vi "Coral Teleop Handler.vi"() -> ()   [LabVIEW 2023]
uses:
  Teleop Util/Coral States.ctl
  Teleop Util/Scoring Setpoint.ctl
  Teleop Util/Scoring Levels.ctl
  <vilib>/Rock Robotics/WPI/Joystick/XBox Axes Indexer.ctl
  <vilib>/Rock Robotics/WPI/Joystick/XBox Buttons Indexer.ctl
  Coral/Implementation/Coral Operations.ctl
  02b96f5f-4aa0-4050-af39-5bf6ce57af74.vi
  ac154037-dd92-4d3b-9487-38ca34f15abd.vi
  41f243a3-b476-470d-886f-9ab9dadf628b.vi
  d73daf83-586d-4580-b12c-c6ead0d00ab0.vi
  <vilib>/Rock Robotics/WPI/Utilities/WPI_GetSetVariantRefNum.vi
  Framework/Robot Global Data.vi
panel:
  in  "Left Rumble":sgl
  out "Final Setpoint":T1=enum."L2"
  in  "Scoring Setpoint":T2=[enum."Trough", enum."L2", enum."L3", enum."L4"]
  out "testing states bz":T3
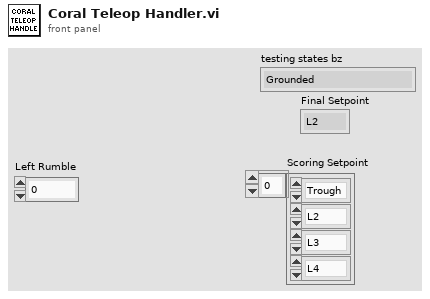
[diagram p1: front panel]
types:
  T1 = typedef "Scoring Levels.ctl" = enum16{"Trough", "L2", "L3", "L4", "Default"}
  T2 = typedef "Scoring Setpoint.ctl" = enum16{"Trough", "L2", "L3", "L4"}[]
  T3 = typedef "Coral States.ctl" = enum16{"Grounded", "Coral Intake", "Scoring Sequence", "Hold Position", "Score", "Manual Override", "Climb Safety Mode"}
  T4 = typedef "XBox Buttons Indexer.ctl" = enum16{"A", "B", "X", "Y", "Left Bumper", "Right Bumper", "Back", "Start", "Left Joystick", "Right Joystick"}
  T5 = typedef "XBox Axes Indexer.ctl" = enum16{"Left X", "Left Y", "Left Trigger", "Right Trigger", "Right X", "Right Y"}
  T6 = typedef "WPI_JoystickDevRef.ctl" = cluster{"Device":T7}
  T7 = typedef "WPI_JoystickDeviceEnum.ctl" = enum16{"USB 0", "USB 1", "USB 2", "USB 3", "USB 4", "USB 5"}
  T8 = typedef "Coral Operations.ctl" = enum16{"Reserve", "Read Current", "Immediate", "Calibrate"}
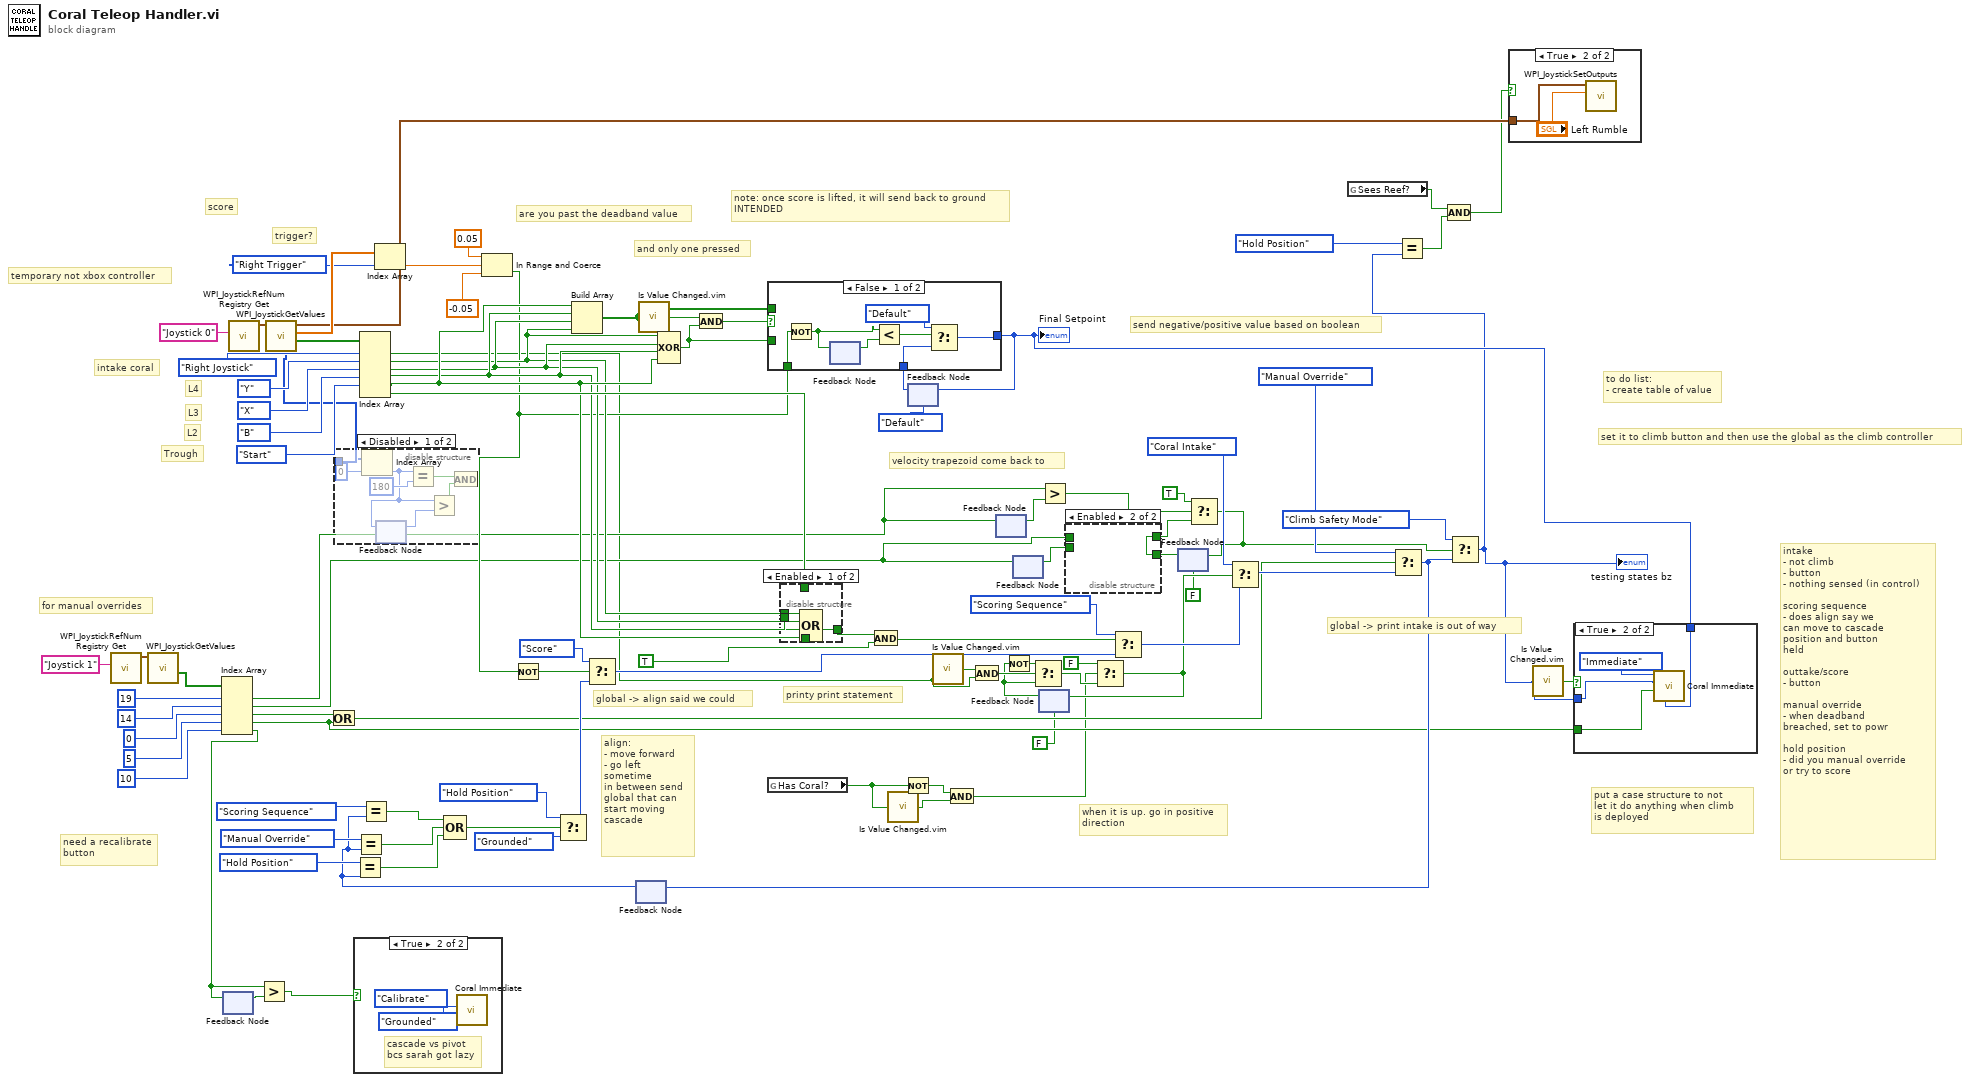
[diagram p0: block diagram]
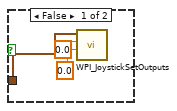
[diagram p2: hidden frame]
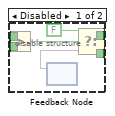
[diagram p4: hidden frame]
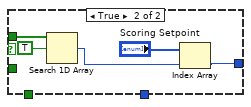
[diagram p8: hidden frame]
diagram:
  # "score"
  # "when it is up. go in positive\ndirection"
  # "send negative/positive value based on boolean"
  # "global -> print intake is out of way"
  # "printy print statement"
  # "set it to climb button and then use the global as the climb controller"
  # "put a case structure to not\nlet it do anything when climb \nis deployed"
  # "note: once score is lifted, it will send back to ground\nINTENDED"
  # "velocity trapezoid come back to"
  # "intake coral"
  # "and only one pressed"
  # "to do list:\n- create table of value"
  # "Trough"
  # "L2"
  # "L3"
  # "L4"
  # "need a recalibrate\nbutton"
  # "align:\n- move forward\n- go left \nsometime \nin between send \nglobal that can \nstart moving \ncascade"
  # "global -> align said we could"
  # "are you past the deadband value"
  # "trigger?"
  # "temporary not xbox controller"
  # "intake\n- not climb\n- button\n- nothing sensed (in control)\n\nscoring sequence\n- does align say we\ncan move to cascade\nposition and button\nheld\n\nouttake/score\n- button\n\nmanual override\n- when deadband\nbreached, set to powr\n\nhold position\n- did you manual override\nor try to score"
  # "for manual overrides"
  n1 = call <vilib>:"WPI_JoystickRefNum Registry Get.vi"("refnum name"="Joystick 1") -> ("JoystickDevRef"=w92:T6)  [unwired: 1 in, 9 out]
  n2 = call <vilib>:"WPI_JoystickGetValues.vi"("JoystickDevRef"=w92) -> ("Buttons"=w90:bool[])  [unwired: 6 in, 4 out]
  n3 = Index Array(array=w90, index #1=19 ("index"), index #2=14 ("index"), index #3=0 ("index"), index #4=5 ("index"), index #5=10 ("index")) -> (element #1=w28:bool, element #2=w29:bool, element #3=w38:bool, element #4=w37:bool, element #5=w32:bool)
  n4 = feedback-in #1(w32) -> ()
  n5 = feedback #1() -> (w45:bool)  [unwired: 1 in]
  n6 = call <vilib>:"WPI_JoystickRefNum Registry Get.vi"("refnum name"="Joystick 0") -> ("JoystickDevRef"=w95:T6)  [unwired: 1 in, 9 out]
  n7 = Greater?(x=w32, y=w45) -> (0:w8:bool)
  n8 = call <vilib>:"WPI_JoystickGetValues.vi"("JoystickDevRef"=w95) -> ("Buttons"=w93:bool[], "Axes"=w77:dbl[], "JoystickDevRef"=w7:T6, "POVs"=w9:i16[])  [unwired: 6 in, 1 out]
  n9 = Or(x=w38, y=w37) -> (x .or. y?=w36:bool)
  n10 = disable-structure shown="Disabled" {
    disable-tunnel: w9 -> [w102 _]
    frame Disabled {
      n11 = Index Array(array=w102, index=0) -> (element=w99:i16)
      n12 = feedback #2() -> (w98:i16)  [unwired: 1 in]
      n13 = feedback-in #2(w99) -> ()
      n14 = Equal?(x=w99, y=i16 180) -> (x = y?=w96:bool)
      n15 = Greater?(x=w99, y=w98) -> (0:w97:bool)
      n16 = And(x=w96, y=w97) -> ()  [unwired: 1 out]
    }
    frame Enabled {
    }
  }
  n17 = case shown="True" w8 {
    frame False {
    }
    frame True {
      # "cascade vs pivot\nbcs sarah got lazy"
      n18 = call "Coral Immediate.vi"("Coral States"=Coral_States."Grounded", "Operation"=Coral_Operations."Calibrate") -> ()  [unwired: 9 in, 1 out]
    }
  }
  n19 = Index Array(array=w93, index #1=XBox_Buttons_Indexer."Right Joystick" ("XBox Buttons"), index #2=XBox_Buttons_Indexer."Y" ("XBox Buttons"), index #3=XBox_Buttons_Indexer."X" ("XBox Buttons"), index #4=XBox_Buttons_Indexer."B" ("XBox Buttons"), index #5=XBox_Buttons_Indexer."Start" ("XBox Buttons")) -> (element #1=w23:bool, element #2=w50:bool, element #3=w51:bool, element #4=w52:bool, element #5=w53:bool, element #6=w54:bool)  [unwired: 1 in]
  n20 = Index Array(array=w77, index=XBox_Axes_Indexer."Right Trigger" ("XBox Axes")) -> (element=w74:dbl)
  n21 = In Range and Coerce(upper limit=0.05 ("lower limit"), x=w74, lower limit=-0.05) -> (In Range?=w39:bool)  [unwired: 1 out]
  n22 = Not(x=w39) -> (.not. x?=w18:bool)
  n23 = Build Array(w53, w52, w51, w50) -> (w66:bool[])
  n24 = feedback #3() -> (w55:T3)  [unwired: 1 in]
  n25 = Equal?(x=Coral_States."Hold Position", y=w55) -> (x = y?=w58:bool)
  n26 = Equal?(x=Coral_States."Manual Override", y=w55) -> (x = y?=w59:bool)
  n27 = Equal?(x=Coral_States."Scoring Sequence", y=w55) -> (x = y?=w60:bool)
  n28 = Compound Arithmetic op=OR(w60, w59, w58) -> (w57:bool)
  n29 = Select(t=Coral_States."Hold Position", s=w57, f=Coral_States."Grounded") -> (s? t:f=w88:T3)
  n30 = Select(t=Coral_States."Score", s=w18, f=w88) -> (s? t:f=w86:T3)
  n31 = call "Is Value Changed.vim"("value"=w66) -> ("changed or first call?"=w67:bool)
  n32 = Compound Arithmetic op=XOR(w50, w51, w52, w53) -> (w64:bool)
  n33 = And(x=w67, y=w64) -> (x .and. y?=w65:bool)
  n34 = global read "Robot Global Data.vi" "Has Coral?"() -> (w17:bool)
  n35 = disable-structure shown="Enabled" {
    disable-tunnel: w50 -> [w109 _]
    disable-tunnel: w51 -> [w108 _]
    disable-tunnel: w52 -> [w107 _]
    disable-tunnel: w53 -> [w106 _]
    disable-tunnel: [w105 w110] -> w62
    disable-tunnel: w54 -> [_ w110]
    frame Enabled {
      n36 = Compound Arithmetic op=OR(w109, w108, w107, w106) -> (w105:bool)
    }
    frame Disabled {
    }
  }
  n37 = And(x=w62, y=TRUE) -> (x .and. y?=w63:bool)
  n38 = call "Is Value Changed.vim"("value"=w17) -> ("changed or first call?"=w16:bool)
  n39 = Not(x=w17) -> (.not. x?=w14:bool)
  n40 = feedback #4(Scoring_Levels."Default" ("t")) -> (w49:T1)
  n41 = case shown="False" w65 {
    tunnel: w66 -> [_ w122]
    tunnel: w64 -> [_ _]
    tunnel: w49 -> [w114 _]
    tunnel: w39 -> [w116 _]
    tunnel: [w112 w118] -> w6
    frame False {
      n42 = Not(x=w116) -> (.not. x?=w111:bool)
      n43 = feedback-in #5(w111) -> ()
      n44 = feedback #5() -> (w115:bool)  [unwired: 1 in]
      n45 = Less?(x=w111, y=w115) -> (x < y?=w117:bool)
      n46 = Select(t=Scoring_Levels."Default", s=w117, f=w114) -> (s? t:f=w112:T1)
    }
    frame True {
      n47 = Search 1D Array(1D array=w122, element=TRUE) -> (index of element=w121:i32)  [unwired: 1 in]
      n48 = Index Array(array="Scoring Setpoint", index=w121) -> (element=w118:enum16{"Trough", "L2", "L3", "L4"})
    }
  }
  "Final Setpoint" <- w6
  n49 = feedback-in #4(w6) -> ()
  n50 = call "Is Value Changed.vim"("value"=w23) -> ("changed or first call?"=w26:bool)
  n51 = And(x=w14, y=w16) -> (x .and. y?=w15:bool)
  n52 = And(x=w26, y=w23) -> (x .and. y?=w27:bool)
  n53 = feedback-in #6(w28) -> ()
  n54 = feedback #6() -> (w44:bool)  [unwired: 1 in]
  n55 = feedback #7() -> (w41:bool)  [unwired: 1 in]
  n56 = feedback-in #7(w29) -> ()
  n57 = feedback #8(FALSE) -> (w25:bool)
  n58 = Not(x=w25) -> (.not. x?=w22:bool)
  n59 = Select(t=w22, s=w27, f=w25) -> (s? t:f=w20:bool)
  n60 = Greater?(x=w28, y=w44) -> (0:w43:bool)
  n61 = Select(t=FALSE, s=w15, f=w20) -> (s? t:f=w21:bool)
  n62 = feedback-in #8(w21) -> ()
  n63 = Select(t=Coral_States."Scoring Sequence", s=w63, f=w86) -> (s? t:f=w85:T3)
  n64 = feedback #9(FALSE) -> (w10:bool)
  n65 = disable-structure shown="Enabled" {
    disable-tunnel: [w128 w129] -> w13
    disable-tunnel: w41 -> [w126 _]
    disable-tunnel: w29 -> [w123 _]
    disable-tunnel: w10 -> [_ w129]
    frame Disabled {
      n66 = Greater?(x=w123, y=w126) -> (0:w125:bool)
      n67 = feedback #10() -> (w127)  [unwired: 1 in]
      n68 = feedback-in #10() -> ()  [unwired: 1 out]
      n69 = Select(t=FALSE, s=w125, f=w127) -> (s? t:f=w128:bool)
    }
    frame Enabled {
    }
  }
  n70 = Select(t=TRUE, s=w43, f=w13) -> (s? t:f=w12:bool)
  n71 = feedback-in #9(w12) -> ()
  n72 = Select(t=Coral_States."Coral Intake", s=w21, f=w85) -> (s? t:f=w84:T3)
  n73 = global read "Robot Global Data.vi" "Sees Reef?"() -> (w3:bool)
  n74 = Select(t=Coral_States."Manual Override", s=w36, f=w84) -> (s? t:f=w47:T3)
  n75 = feedback-in #3(w47) -> ()
  n76 = Select(t=Coral_States."Climb Safety Mode", s=w12, f=w47) -> (s? t:f=w5:T3)
  "testing states bz" <- w5
  n77 = Equal?(x=Coral_States."Hold Position", y=w5) -> (x = y?=w1:bool)
  n78 = Compound Arithmetic op=AND(w3, w1) -> (w2:bool)
  n79 = case shown="True" w2 {
    tunnel: w7 -> [w132 w134]
    frame False {
      n80 = call <vilib>:"WPI_JoystickSetOutputs.vi"("Right Rumble"=sgl 0.0, "Left Rumble"=sgl 0.0, "JoystickDevRef"=w132) -> ()  [unwired: 7 in, 2 out]
    }
    frame True {
      n81 = call <vilib>:"WPI_JoystickSetOutputs.vi"("Left Rumble"="Left Rumble", "JoystickDevRef"=w134) -> ()  [unwired: 8 in, 2 out]
    }
  }
  n82 = call "Is Value Changed.vim"("value"=w5) -> ("changed or first call?"=w48:bool)
  n83 = case shown="True" w48 {
    tunnel: w6 -> [_ w137]
    tunnel: w5 -> [_ w136]
    tunnel: w37 -> [_ w135]
    frame False {
    }
    frame True {
      n84 = call "Coral Immediate.vi"("Setpoint State"=w137, "Confirm or Negate"=w135, "Coral States"=w136, "Operation"=Coral_Operations."Immediate") -> ()  [unwired: 7 in, 1 out]
    }
  }
